vi "SM_S700_Serial_String_to_gasvalues.vi"(8 "error in (no error)":errorcluster, 10 "String":string, 11 "initial scan location in":u32) -> (0 "error out":errorcluster, 1 "co2":dbl, 2 "ch4":dbl, 3 "h2":dbl)   [LabVIEW 2011]
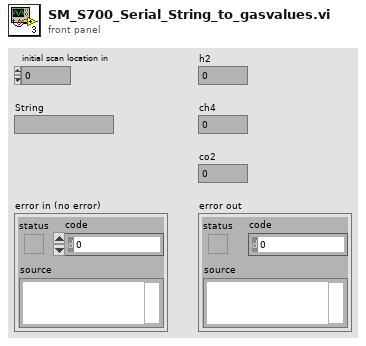
[diagram p1: front panel]
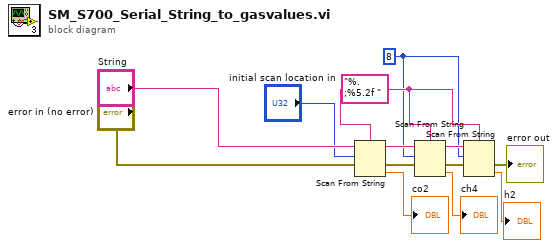
[diagram p0: block diagram]
diagram:
  w1 = u32 8 ("initial scan location 3")
  w8 = "%.;%5.2f " ("format string")
  n1 = Scan From String(format string=w8, input string="String", initial scan location="initial scan location in", error in="error in (no error)") -> (remaining string=w11:string, error out=w10:errorcluster, output 1=→"co2":dbl)  [unwired: 1 in, 1 out]
  n2 = Scan From String(format string=w8, input string=w11, initial scan location=w1, error in=w10) -> (remaining string=w9:string, error out=w4:errorcluster, output 1=→"ch4":dbl)  [unwired: 1 in, 1 out]
  n3 = Scan From String(format string=w8, input string=w9, initial scan location=w1, error in=w4) -> (error out=→"error out":errorcluster, output 1=→"h2":dbl)  [unwired: 1 in, 2 out]
